vi "Teleop.vi"(10 "Match Info":T1={"Autonomous Elapsed Seconds"=0.0, "TeleOp Elapsed Seconds"=0.0, "Disabled Elapsed Seconds"=0.0, "Visited Autonomous"=FALSE, "Visited TeleOp"=FALSE, "Visited Disabled"=FALSE, "Autonomous Settings"={"Autonomous Style"=enum."Independent", "VI Refnum"=refnum}}, 11 "Call Context":T2) -> ()   [LabVIEW 2020]
doc: "This VI is called for each enabled TeleOp packet received from the DS. It is typically used to read from joysticks and other inputs and update I/O or setpoints for timed control loops. It should complete and return within 20 milliseconds or risk missing DS packets."
uses:
  <vilib>/Rock Robotics/WPI/DriverStation/WPI_DriverStationDerivedRobotMode.ctl
  <vilib>/Rock Robotics/WPI/DriverStation/WPI_DriverStationMatch Info.ctl
  <vilib>/Rock Robotics/WPI/Utilities/WPI_GetSetVariantRefNum.vi
  <vilib>/Rock Robotics/Network Tables/NT Write Boolean Array.vi
  <vilib>/Rock Robotics/Network Tables/NT Write Numeric Array.vi
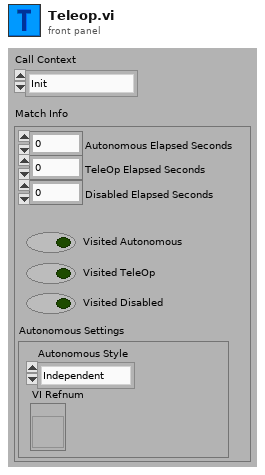
[diagram p1: front panel]
types:
  T1 = typedef "WPI_DriverStationMatch Info.ctl" = cluster{"Autonomous Elapsed Seconds":dbl, "TeleOp Elapsed Seconds":dbl, "Disabled Elapsed Seconds":dbl, "Visited Autonomous":bool, "Visited TeleOp":bool, "Visited Disabled":bool, "Autonomous Settings":cluster{"Autonomous Style":enum16{"Iterative", "Independent"}, "VI Refnum":refnum<vi>}}
  T2 = typedef "WPI_DriverStationDerivedRobotMode.ctl" = enum16{"Init", "Execute", "Stop"}
  T3 = typedef "WPI_JoystickDevRef.ctl" = cluster{"Device":T4}
  T4 = typedef "WPI_JoystickDeviceEnum.ctl" = enum16{"USB 0", "USB 1", "USB 2", "USB 3", "USB 4", "USB 5"}
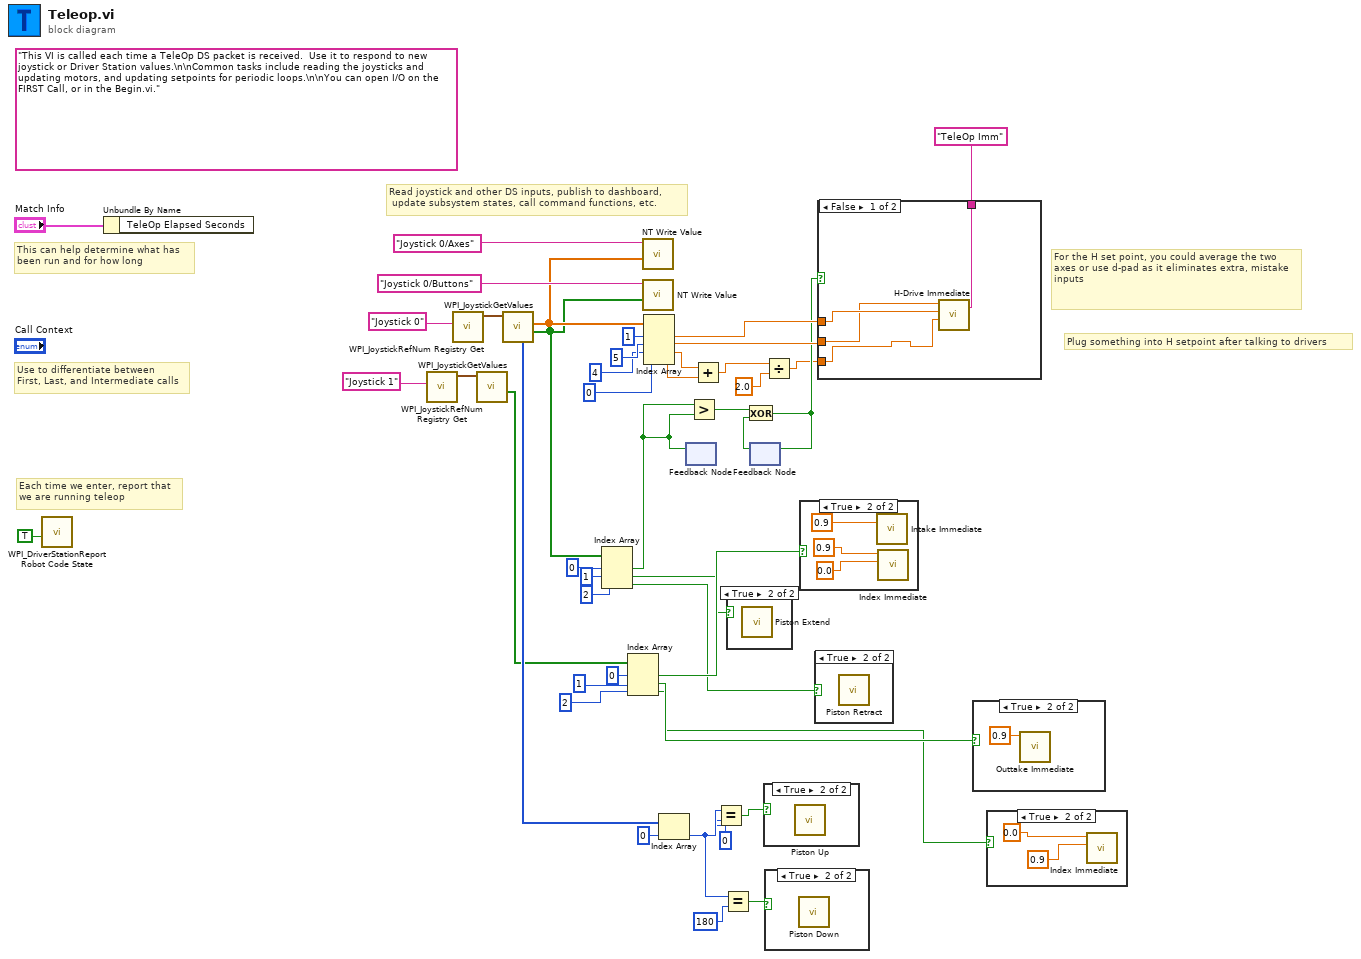
[diagram p0: block diagram]
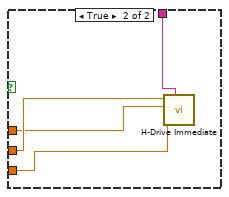
[diagram p9: hidden frame]
diagram:
  (unwired) "This VI is called each time a TeleOp DS packet is received.  Use it to respond to new joystick or Driver Station values.\n\nCommon tasks include reading the joysticks and updating motors, and updating setpoints for periodic loops.\n\nYou can open I/O on the FIRST Call, or in the Begin.vi."
  # "Plug something into H setpoint after talking to drivers"
  # "For the H set point, you could average the two axes or use d-pad as it eliminates extra, mistake inputs"
  # "Read joystick and other DS inputs, publish to dashboard,\n update subsystem states, call command functions, etc."
  # "Each time we enter, report that\nwe are running teleop"
  # "Use to differentiate between\nFirst, Last, and Intermediate calls"
  # "This can help determine what has\nbeen run and for how long"
  n1 = call <vilib>:"WPI_DriverStationReport Robot Code State.vi"("TeleOp"=TRUE ("Autonomous")) -> ()  [unwired: 10 in, 1 out]
  n2 = Unbundle By Name("Match Info") -> ()  [unwired: 1 out]
  n3 = call <vilib>:"WPI_JoystickRefNum Registry Get.vi"("refnum name"="Joystick 1") -> ("JoystickDevRef"=w26:T3)  [unwired: 1 in, 9 out]
  n4 = call <vilib>:"WPI_JoystickRefNum Registry Get.vi"("refnum name"="Joystick 0") -> ("JoystickDevRef"=w42:T3)  [unwired: 1 in, 9 out]
  n5 = call <vilib>:"WPI_JoystickGetValues.vi"("JoystickDevRef"=w26) -> ("Buttons"=w13:bool[])  [unwired: 6 in, 4 out]
  n6 = call <vilib>:"WPI_JoystickGetValues.vi"("JoystickDevRef"=w42) -> ("Buttons"=w38:bool[], "Axes"=w40:dbl[], "POVs"=w29:i16[])  [unwired: 6 in, 2 out]
  n7 = Index Array(array=w38, index #1=0 ("index"), index #2=1 ("index"), index #3=2 ("index")) -> (element #1=w18:bool, element #2=w2:bool, element #3=w1:bool)
  n8 = Index Array(array=w13, index #1=0 ("index"), index #2=1 ("index"), index #3=2 ("index")) -> (element #1=w11:bool, element #2=w9:bool, element #3=w7:bool)
  n9 = call-poly <vilib>:"NT Write Value.vi"("Numeric Array"=w40, "Name"="Joystick 0/Axes") -> ()  [unwired: 9 in, 1 out]
  n10 = call-poly <vilib>:"NT Write Value.vi"("Boolean Array"=w38, "Name"="Joystick 0/Buttons") -> ()  [unwired: 9 in, 1 out]
  n11 = Index Array(array=w40, index #1=1 ("index"), index #2=5 ("index"), index #3=4, index #4=0 ("index")) -> (element #1=w35:dbl, element #2=w34:dbl, element #3=w22:dbl, element #4=w21:dbl)
  n12 = Index Array(array=w29, index=0) -> (element=w17:i16)
  n13 = feedback-in #1(w18) -> ()
  n14 = feedback #1() -> ()  [unwired: 2 in]
  n15 = Greater?(x=w18, y=w18) -> (0:w33:bool)
  n16 = Add(x=w22, y=w21) -> (x+y=w20:dbl)
  n17 = Equal?(x=w17, y=0) -> (x = y?=w6:bool)
  n18 = Equal?(x=w17, y=180) -> (x = y?=w5:bool)
  n19 = case shown="True" w2 {
    frame False {
    }
    frame True {
      n20 = call "Piston Extend.vi"() -> ()  [unwired: 11 in, 1 out]
    }
  }
  n21 = feedback #2() -> (w32:bool)  [unwired: 1 in]
  n22 = Exclusive Or(1:w32, 2:w33) -> (0:w31:bool)
  n23 = feedback-in #2(w31) -> ()
  n24 = Divide(x=w20, y=2.0) -> (x/y=w23:dbl)
  n25 = case shown="True" w6 {
    frame False {
    }
    frame True {
      n26 = call "Piston Up.vi"() -> ()  [unwired: 11 in, 1 out]
    }
  }
  n27 = case shown="True" w5 {
    frame False {
    }
    frame True {
      n28 = call "Piston Down.vi"() -> ()  [unwired: 11 in, 1 out]
    }
  }
  n29 = case shown="True" w11 {
    frame False {
    }
    frame True {
      n30 = call "Intake Immediate.vi"("Setpoint"=0.9) -> ()  [unwired: 10 in, 1 out]
      n31 = call "Index Immediate.vi"("Feeder Motor Setpoint"=0.0, "Indexer Motor Setpoint"=0.9 ("Setpoint")) -> ()  [unwired: 9 in, 1 out]
    }
  }
  n32 = case shown="True" w1 {
    frame False {
    }
    frame True {
      n33 = call "Piston Retract.vi"() -> ()  [unwired: 11 in, 1 out]
    }
  }
  n34 = case shown="False" w31 {
    tunnel: w35 -> [w50 w53]
    tunnel: w34 -> [w49 w54]
    tunnel: "TeleOp Imm" ("Description") -> [w52 w56]
    tunnel: w23 -> [w51 w55]
    frame False {
      n35 = call "H-Drive Immediate.vi"("Description"=w52, "H Setpoint"=w51, "Right Setpoint"=w50, "Left Setpoint"=w49) -> ()  [unwired: 7 in, 1 out]
    }
    frame True {
      n36 = call "H-Drive Immediate.vi"("Description"=w56, "H Setpoint"=w55, "Right Setpoint"=w53, "Left Setpoint"=w54) -> ()  [unwired: 7 in, 1 out]
    }
  }
  n37 = case shown="True" w9 {
    frame False {
    }
    frame True {
      n38 = call "Outtake Immediate.vi"("Setpoint"=0.9) -> ()  [unwired: 10 in, 1 out]
    }
  }
  n39 = case shown="True" w7 {
    frame False {
    }
    frame True {
      n40 = call "Index Immediate.vi"("Feeder Motor Setpoint"=0.9, "Indexer Motor Setpoint"=0.0) -> ()  [unwired: 9 in, 1 out]
    }
  }
